vi "Place_Missed_Tracks-1.vi"(4 "[IN] Missed Start Pos":i32[](array[numeric]), 6 "[IN] Missed Dot Status":i16[][](array[numeric]), 8 "error IN":errorcluster, 9 "[IN] Missed tracks":dbl[][](array[numeric]), 11 "[IN] Before Pro\ncessing Tracks":T1(array[cluster])) -> (0 "error OUT":errorcluster, 3 "[OUT] Processed Tracks":T1(array[cluster]))   [LabVIEW 2013]
panel:
  out "Number of assignments":u8
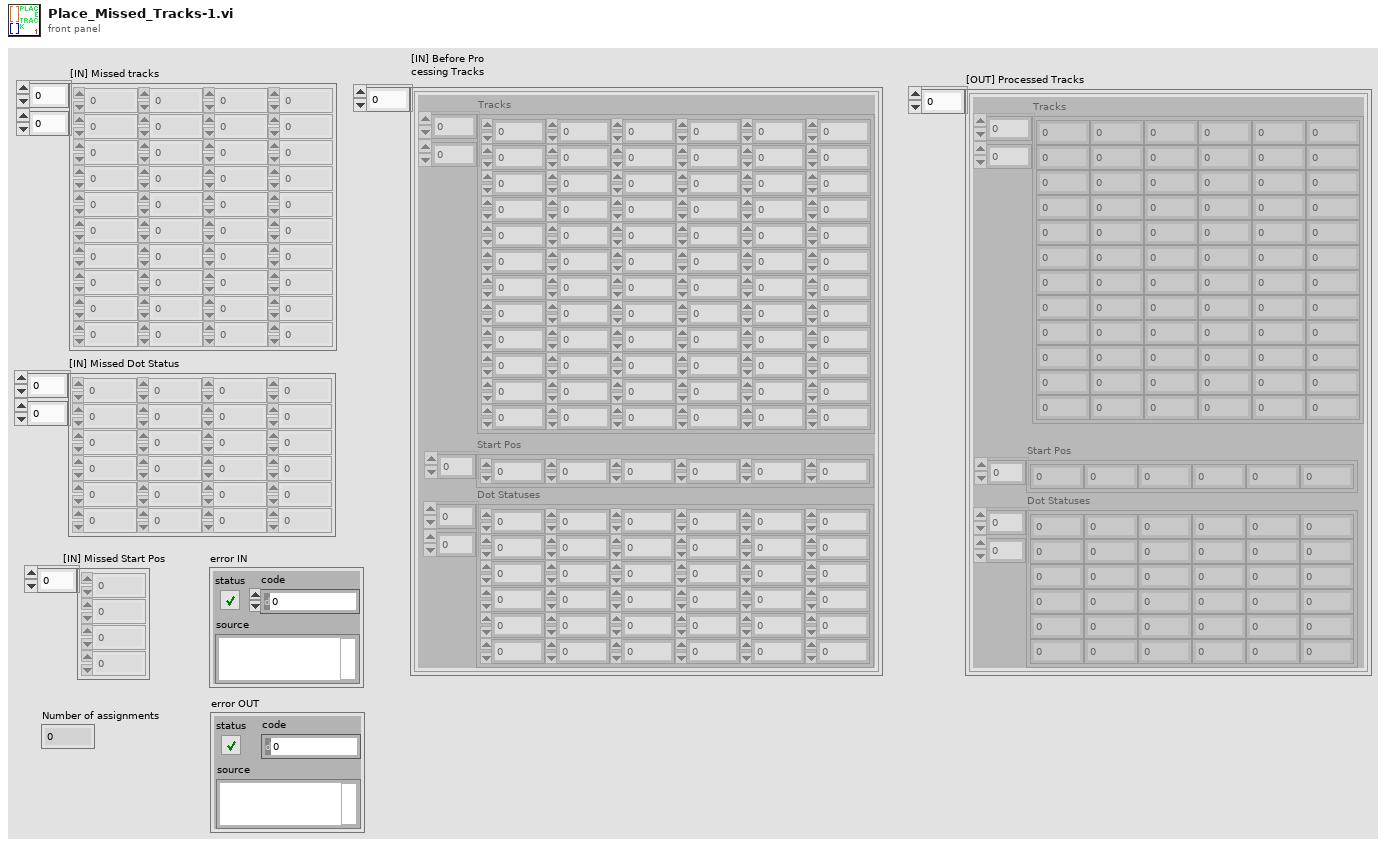
[diagram p1: front panel]
types:
  T1 = cluster{"Tracks":dbl[][], "Start Pos":i32[], "Dot Statuses":i16[][]}[]
  T2 = cluster{"Tracks":dbl[][], "Start Pos":i32[], "Dot Statuses":i16[][]}
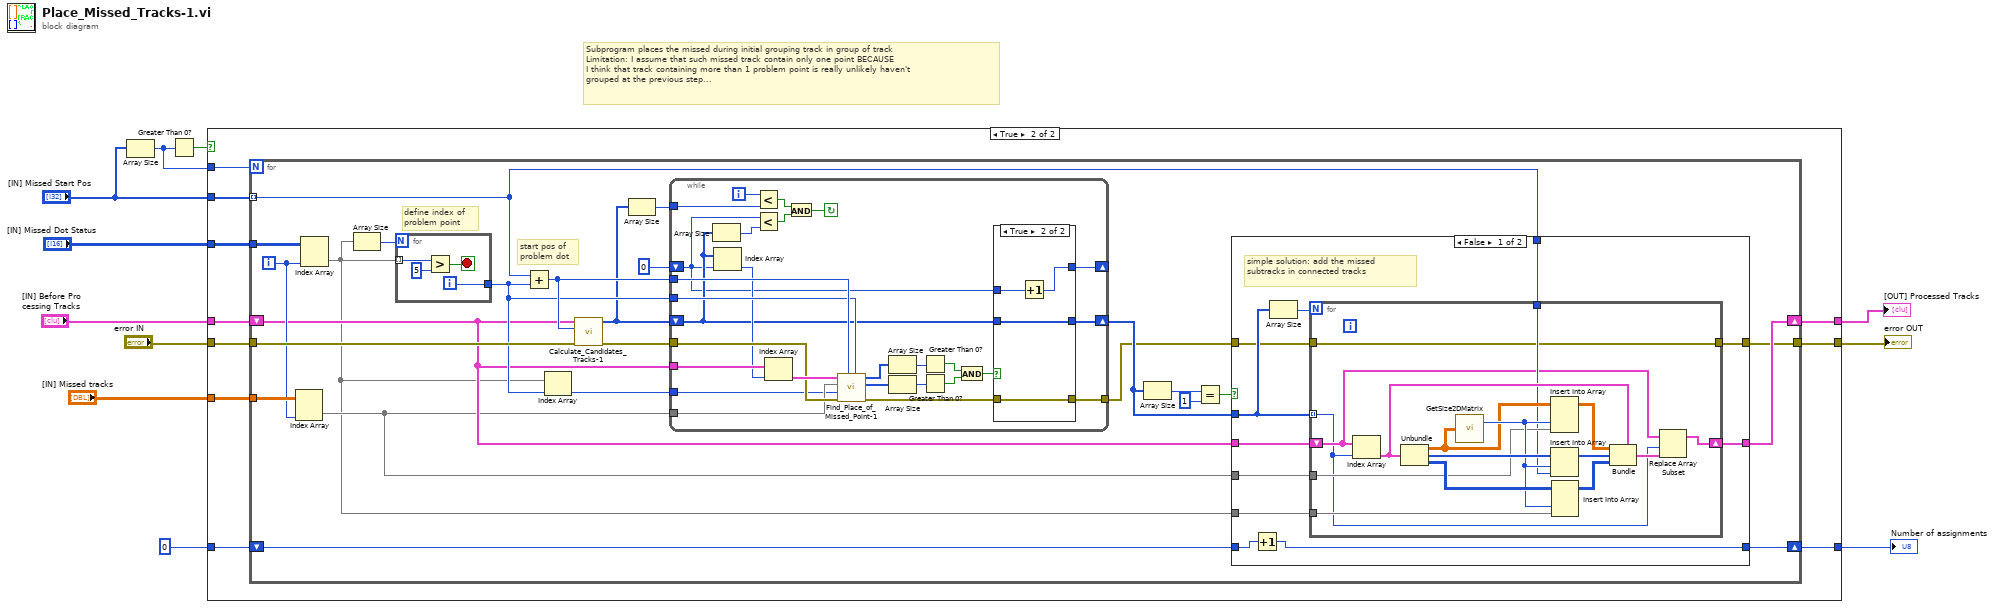
[diagram p0: block diagram]
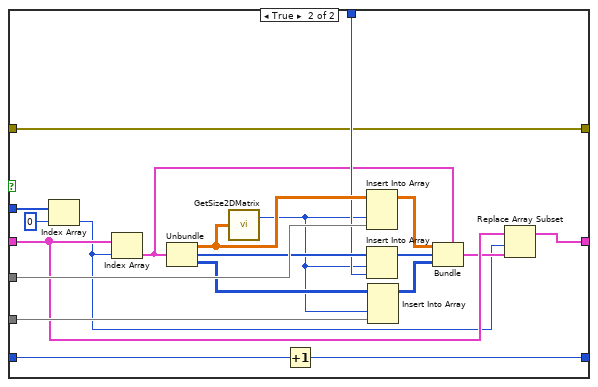
[diagram p3: hidden frame]
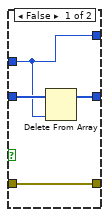
[diagram p4: hidden frame]
diagram:
  # "Subprogram places the missed during initial grouping track in group of track\nLimitation: I assume that such missed track contain only one point BECAUSE\nI think that track containing more than 1 problem point is really unlikely haven't \ngrouped at the previous step..."
  n1 = Array Size(array="[IN] Missed Start Pos") -> (size(s)=w10:i32)
  n2 = Greater Than 0?(x=w10) -> (x > 0?=w11:bool)
  n3 = case shown="True" w11 {
    tunnel: w10 -> [_ w24]
    tunnel: "[IN] Missed Start Pos" -> [_ w23]
    tunnel: "[IN] Before Pro\ncessing Tracks" -> [w14 w22]
    tunnel: "[IN] Missed Dot Status" -> [_ w21]
    tunnel: "error IN" -> [w13 w20]
    tunnel: "[IN] Missed tracks" -> [_ w19]
    tunnel: [w14 w18] -> w3
    tunnel: [w13 w17] -> w4
    tunnel: u8 0 -> [w12 w16]
    tunnel: [w12 w15] -> w1
    frame False {
    }
    frame True {
      n4 = for {
        N: w24 -> [_]
        tunnel: w23 -> [w31] mode=indexing
        tunnel: w21 -> [w49]
        tunnel: w20 -> [w47]
        tunnel: w19 -> [w44]
        shift-right: [w29] -> w18
        shift-left: w22 -> [w34]
        tunnel: [w27] -> w17
        shift-right: [w25] -> w15
        shift-left: w16 -> [w26]
        i -> [w43]
        # "start pos of \nproblem dot"
        # "define index of \nproblem point"
        n5 = Index Array(array=w44, index (col)=w43) -> (element=w32:dbl[])  [unwired: 1 in]
        n6 = Index Array(array=w49, index (col)=w43) -> (element=w30:i16[])  [unwired: 1 in]
        n7 = Array Size(array=w30) -> (size(s)=w48:i32)
        n8 = for {
          N: w48 -> [_]
          tunnel: w30 -> [w135] mode=indexing
          tunnel: [w132] -> w42
          i -> [w132]
          stop <- w133 stop-if-true
          n9 = Greater?(x=w135, y=i16 5) -> (0:w133:bool)
        }
        n10 = Add(x=w31, y=w42) -> (x+y=w45:i32)
        n11 = Index Array(array=w30, index=w42) -> (element=w41:i16)
        n12 = call "Calculate_Candidates_Tracks-1.vi"("error IN"=w47, "[IN] Start Pos of\nMissed Pr Dot"=w45, "[IN] Before Pro\ncessing Tracks"=w34) -> ("error OUT"=w46:errorcluster, "[OUT] Indicies of \ngroup candidates"=w40:i32[])  [unwired: 3 in]
        n13 = Array Size(array=w40) -> (size(s)=w39:i32)
        n14 = while {
          tunnel: w34 -> [w123]
          tunnel: w46 -> [w121]
          tunnel: w45 -> [w120]
          tunnel: w42 -> [w119]
          tunnel: w32 -> [w118]
          tunnel: w41 -> [w117]
          shift-right: [w109] -> w33
          shift-left: w40 -> [w105]
          tunnel: w39 -> [w107]
          shift-right: [w99] -> _
          shift-left: 0 -> [w100]
          tunnel: [w97] -> w28
          i -> [w108]
          stop <- w101 continue-if-true
          n15 = Array Size(array=w105) -> (size(s)=w104:i32)
          n16 = Index Array(array=w105, index=w100) -> (element=w106:i32)
          n17 = Less?(x=w108, y=w107) -> (x < y?=w103:bool)
          n18 = Less?(x=w100, y=w104) -> (x < y?=w102:bool)
          n19 = Index Array(array=w123, index=w106) -> (element=w122:T2)
          n20 = And(x=w103, y=w102) -> (x .and. y?=w101:bool)
          n21 = call "Find_Place_of_Missed_Point-1.vi"("[IN] Index of problem\ndisplacement inside track"=w119, "[IN] Time Point of Mi\nssed Problem Dot"=w120, "error IN"=w121, "[IN] Dot Status"=w117, "[IN] Missed track"=w118, "[IN] Track group"=w122) -> ("error OUT"=w98:errorcluster, "[OUT] Index of \nconnected dots\ninside the track"=w115:i32[], "[OUT] Index of connected\ntracks with problem dot"=w116:i32[])  [unwired: 1 in]
          n22 = Array Size(array=w116) -> (size(s)=w114:i32)
          n23 = Array Size(array=w115) -> (size(s)=w113:i32)
          n24 = Greater Than 0?(x=w114) -> (x > 0?=w112:bool)
          n25 = Greater Than 0?(x=w113) -> (x > 0?=w111:bool)
          n26 = And(x=w112, y=w111) -> (x .and. y?=w110:bool)
          n27 = case shown="True" w110 {
            tunnel: w105 -> [w127 w131]
            tunnel: [w126 w131] -> w109
            tunnel: w100 -> [w125 w130]
            tunnel: [w125 w129] -> w99
            tunnel: w98 -> [w124 w128]
            tunnel: [w124 w128] -> w97
            frame False {
              n28 = Delete From Array(array=w127, index=w125) -> (array with subset deleted=w126:i32[])  [unwired: 1 in, 1 out]
            }
            frame True {
              n29 = Increment(x=w130) -> (x+1=w129:i32)
            }
          }
        }
        n30 = Array Size(array=w33) -> (size(s)=w37:i32)
        n31 = Equal?(x=w37, y=1) -> (x = y?=w35:bool)
        n32 = case shown="False" w35 {
          tunnel: w34 -> [w57 w83]
          tunnel: w33 -> [w59 w96]
          tunnel: w32 -> [w53 w93]
          tunnel: w31 -> [w52 w91]
          tunnel: w30 -> [w51 w88]
          tunnel: [w54 w80] -> w29
          tunnel: w28 -> [w58 w79]
          tunnel: [w50 w79] -> w27
          tunnel: w26 -> [w56 w78]
          tunnel: [w55 w77] -> w25
          frame False {
            # "simple solution: add the missed \nsubtracks in connected tracks"
            n33 = Increment(x=w56) -> (x+1=w55:u8)
            n34 = Array Size(array=w59) -> (size(s)=w60:i32)
            n35 = for {
              N: w60 -> [_]
              tunnel: w59 -> [w62] mode=indexing
              tunnel: w58 -> [w61]
              shift-right: [w63] -> w54
              shift-left: w57 -> [w65]
              tunnel: w53 -> [w70]
              tunnel: w52 -> [w67]
              tunnel: w51 -> [w66]
              tunnel: [w61] -> w50
              n36 = Index Array(array=w65, index=w62) -> (element=w71:T2)
              n37 = Unbundle(w71) -> ("Tracks"=w69:dbl[][], "Start Pos"=w76:i32[], "Dot Statuses"=w75:i16[][])
              n38 = call "GetSize2DMatrix.vi"("Array IN (2D)"=w69) -> ("# Cols"=w74:i32)  [unwired: 1 out]
              n39 = Insert Into Array(array=w69, index (col)=w74, new element=w70) -> (w68:dbl[][])  [unwired: 1 in]
              n40 = Insert Into Array(array=w76, index=w74, new element=w67) -> (w73:i32[])
              n41 = Insert Into Array(array=w75, index (col)=w74, new element=w66) -> (w72:i16[][])  [unwired: 1 in]
              n42 = Bundle(cluster=w71, "Tracks"=w68, "Start Pos"=w73, "Dot Statuses"=w72) -> (w64:T2)
              n43 = Replace Array Subset(array=w65, new element=w64, index=w62) -> (w63:T1)
            }
          }
          frame True {
            n44 = Index Array(array=w96, index=0) -> (element=w81:i32)
            n45 = Index Array(array=w83, index=w81) -> (element=w87:T2)
            n46 = Unbundle(w87) -> ("Tracks"=w94:dbl[][], "Start Pos"=w92:i32[], "Dot Statuses"=w90:i16[][])
            n47 = call "GetSize2DMatrix.vi"("Array IN (2D)"=w94) -> ("# Cols"=w89:i32)  [unwired: 1 out]
            n48 = Increment(x=w78) -> (x+1=w77:u8)
            n49 = Insert Into Array(array=w94, index (col)=w89, new element=w93) -> (w86:dbl[][])  [unwired: 1 in]
            n50 = Insert Into Array(array=w92, index=w89, new element=w91) -> (w85:i32[])
            n51 = Insert Into Array(array=w90, index (col)=w89, new element=w88) -> (w84:i16[][])  [unwired: 1 in]
            n52 = Bundle(cluster=w87, "Tracks"=w86, "Start Pos"=w85, "Dot Statuses"=w84) -> (w82:T2)
            n53 = Replace Array Subset(array=w83, new element=w82, index=w81) -> (w80:T1)
          }
        }
      }
    }
  }
  "error OUT" <- w4
  "[OUT] Processed Tracks" <- w3
  "Number of assignments" <- w1
